vi "Make Name.vi"() -> (0 "Actor Name":string)   [LabVIEW 2020, in "Simple Chat.lvlib" / "Simple Chat.lvclass"]
uses:
  Simple Chat.lvclass
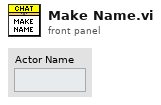
[diagram p1: front panel]
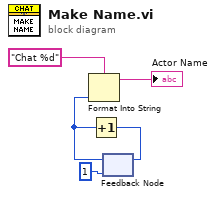
[diagram p0: block diagram]
diagram:
  n1 = feedback #1(1) -> (w3:i32)
  n2 = Format Into String(format string="Chat %d", w3) -> (resulting string=→"Actor Name":string)  [unwired: 2 in, 1 out]
  n3 = Increment(x=w3) -> (x+1=w2:i32)
  n4 = feedback-in #1(w2) -> ()
